vi "Update Data.vi"(0 "data in":T2, 1 "block size (elements)":i32, 2 "(empty) elements remaining":u32, 3 "command":refnum<notifier>, 4 "writing?":bool, 5 "error in (no error)":errorcluster, 8 "pending blocks in host buffer":i32) -> (14 "data out":T2, 15 "status":T1, 16 "preview size (elements)":i32, 17 "reopen file":bool, 18 "reopen total count (elements)":i64, 19 "error out":errorcluster)   [LabVIEW 2021, in "Disk Streaming.lvclass"]
doc: "Updates the disk streaming data with the transfer of a block, processes commands and prepares the status information.\n\nInputs:\n\n<B>data in</B>: Disk streaming data input.\n\n<B>block size (elements)</B>: The number of elements transferred in the block.\n\n<B>(empty) elements remaining</B>: When streaming from device to disk, set this input to the number of additional elements remaining in the host DMA buffer that are available for reading. When streaming from disk to device, set this input to the number of additional empty elements remaining in the host DMA buffer that are available for writing. This input is used only in the calculation of the Host DMA buffer utilization status.\n\n<B>command</B>: Reference to a notifier containing the last command.\n\n<B>writing?</B>: Set this input to true when streaming from device to disk, set this input to false when streaming from disk to device.\n\n<B>pending blocks in host buffer</B>: The number of the last blocks (including the current block transferring the <B>block size</B> elements) whose size is to be added to the Host DMA buffer utilization status. This input is used only in the calculation of the Host DMA buffer utilization status.\n\nOutputs:\n\n<B>data out</B>: Disk streaming data output.\n\n<B>status</B>: The disk streaming status. The status is not complete, this VI does not set the following elements in the status cluster: <B>Disk pending async operations</B> and <B>preview data</B>.\n\n<B>preview size (elements)</B>: The number of elements to use from the last block as the preview data.\n\n<B>reopen file</B>: A true on this output signals that the file should be reopened before reading the next block from it.\n\n<B>reopen total count (elements)</B>: The total number of elements to read from the file on a reopen to complete the streaming operation or until the next reopening of the file."
uses:
  Disk Streaming.lvclass
  Command.ctl
  Data.ctl
  Public/IO mode.ctl
  Status.ctl
  <vilib>/Utility/error.llb/Error Cluster From Error Code.vi
  <vilib>/ErrorRing/Error Ring.xnode
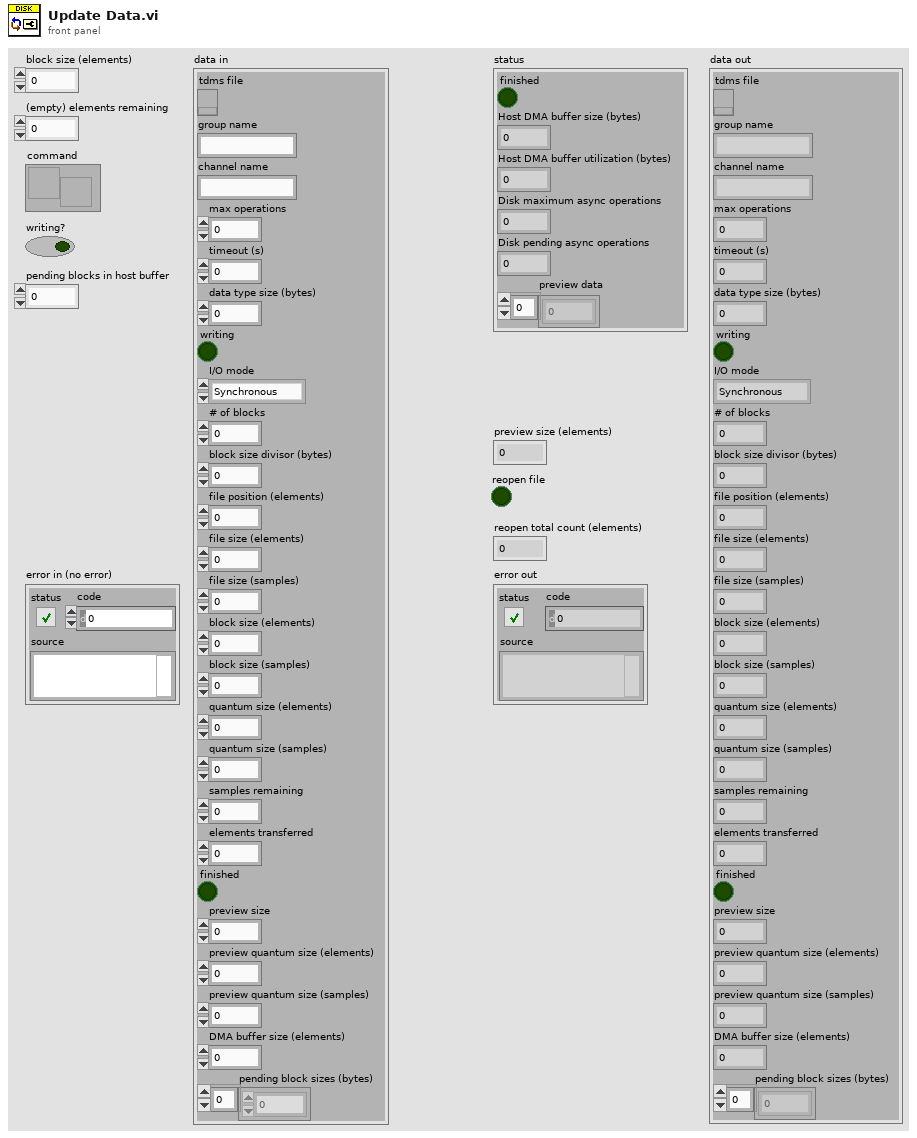
[diagram p1: front panel]
types:
  T1 = typedef "Disk Streaming.lvclass/Status.ctl" = cluster{"finished":bool, "Host DMA buffer size (bytes)":u64, "Host DMA buffer utilization (bytes)":u64, "Disk maximum async operations":u32, "Disk pending async operations":u32, "preview data":i16[]}
  T2 = typedef "Disk Streaming.lvclass/Data.ctl" = cluster{"tdms file":refnum<k34>, "group name":string, "channel name":string, "max operations":u32, "timeout (s)":dbl, "data type size (bytes)":u64, "writing":bool, "I/O mode":T3, "# of blocks":u32, "block size divisor (bytes)":u32, "file position (elements)":u64, "file size (elements)":i64, "file size (samples)":i64, "block size (elements)":u64, "block size (samples)":u64, "quantum size (elements)":u64, "quantum size (samples)":u64, "samples remaining":i64, "elements transferred":u64, "finished":bool, "preview size":i32, "preview quantum size (elements)":u64, "preview quantum size (samples)":u64, "DMA buffer size (elements)":u32, "pending block sizes (bytes)":u64[]}
  T3 = typedef "Disk Streaming.lvclass/IO mode.ctl" = enum16{"Synchronous", "Asynchronous", "Data Reference"}
  T4 = typedef "Disk Streaming.lvclass/Command.ctl" = cluster{"preview size":i32}
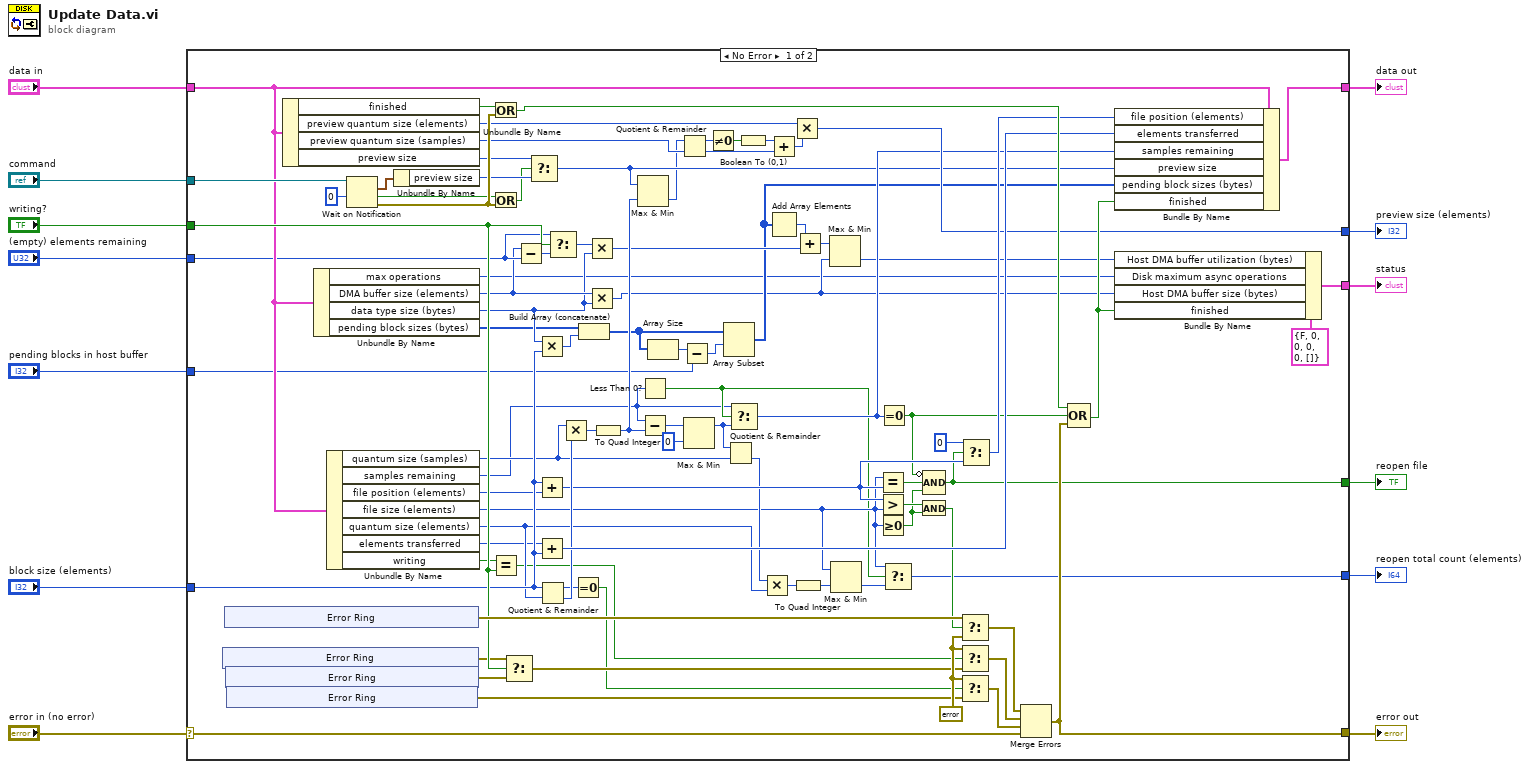
[diagram p0: block diagram]
diagram:
  n1 = case shown="No Error" "error in (no error)" {
    selector: "error in (no error)" -> [w78 w123]
    tunnel: "(empty) elements remaining" -> [w60 _]
    tunnel: "command" -> [w86 _]
    tunnel: [w83 w124] -> w11
    tunnel: "data in" -> [w61 w124]
    tunnel: [w89 w123] -> w8
    tunnel: "block size (elements)" -> [w44 _]
    tunnel: [w77 _] -> w6
    tunnel: "writing?" -> [w93 _]
    tunnel: [w63 _] -> w4
    tunnel: [w50 _] -> w3
    tunnel: "pending blocks in host buffer" -> [w41 _]
    tunnel: [w23 _] -> w1
    frame No Error {
      w101 = errorcluster {"status"=FALSE, "code"=0, "source"=""} ("t")
      n2 = xnode "Error Ring"() -> ("error out"=w88:errorcluster)
      n3 = xnode "Error Ring"() -> ("error out"=w100:errorcluster)
      n4 = xnode "Error Ring"() -> ("error out"=w87:errorcluster)
      n5 = xnode "Error Ring"() -> ("error out"=w99:errorcluster)
      n6 = Unbundle By Name(w61) -> ("finished"=w74:bool, "preview quantum size (elements)"=w51:u64, "preview quantum size (samples)"=w52:u64, "preview size"=w73:i32)
      n7 = Unbundle By Name(w61) -> ("max operations"=w14:u32, "DMA buffer size (elements)"=w58:u32, "data type size (bytes)"=w45:u64, "pending block sizes (bytes)"=w38:u64[])
      n8 = Unbundle By Name(w61) -> ("quantum size (samples)"=w31:u64, "samples remaining"=w18:i64, "file position (elements)"=w21:u64, "file size (elements)"=w25:i64, "quantum size (elements)"=w29:u64, "elements transferred"=w19:u64, "writing"=w20:bool)
      n9 = Wait on Notification(notifier=w86, timeout in ms (-1)=0) -> (notification=w84:T4, timed out?=w48:bool, error out=w95:errorcluster)  [unwired: 2 in, 1 out]
      n10 = Unbundle By Name(w84) -> ("preview size"=w72:i32)
      n11 = Or(x=w74, y=w95) -> (x .or. y?=w97:bool)
      n12 = Or(x=w48, y=w95) -> (x .or. y?=w47:bool)
      n13 = Equal?(x=w20, y=w93) -> (x = y?=w22:bool)
      n14 = Select(t=w88, s=w93, f=w87) -> (s? t:f=w98:errorcluster)
      n15 = Subtract(x=w58, y=w60) -> (x-y=w62:u32)
      n16 = Select(t=w73, s=w47, f=w72) -> (s? t:f=w16:i32)
      n17 = Multiply(x=w45, y=w44) -> (x*y=w43:u64)
      n18 = Add(x=w44, y=w21) -> (x+y=w68:u64)
      n19 = Add(x=w19, y=w44) -> (x+y=w94:u64)
      n20 = Quotient & Remainder(x=w44, y=w29) -> (x-y*floor(x/y)=w65:u64, floor(x/y)=w82:u64)
      n21 = Select(t=w60, s=w93, f=w62) -> (s? t:f=w59:u32)
      n22 = Multiply(x=w31, y=w82) -> (x*y=w17:u64)
      n23 = Equal To 0?(x=w65) -> (x = 0?=w91:bool)
      n24 = Build Array (concatenate)(w38, w43) -> (w39:u64[])
      n25 = Multiply(x=w59, y=w45) -> (x*y=w49:u64)
      n26 = Multiply(x=w58, y=w45) -> (x*y=w33:u64)
      n27 = To Quad Integer(1:w17) -> (0:w102:i64)
      n28 = Max & Min(x=w16, y=w102) -> (min(x,y)=w15:i64)  [unwired: 1 out]
      n29 = Less Than 0?(x=w18) -> (x < 0?=w24:bool)
      n30 = Subtract(x=w18, y=w102) -> (x-y=w81:i64)
      n31 = Array Size(array=w39) -> (size(s)=w42:i32)
      n32 = Quotient & Remainder(x=w15, y=w52) -> (x-y*floor(x/y)=w53:u64, floor(x/y)=w56:u64)
      n33 = Subtract(x=w42, y=w41) -> (x-y=w40:i32)
      n34 = Max & Min(x=w81, y=i64 0) -> (max(x,y)=w32:i64)  [unwired: 1 out]
      n35 = Not Equal To 0?(x=w53) -> (x != 0?=w54:bool)
      n36 = Array Subset(array=w39, index=w40) -> (w37:u64[])  [unwired: 1 in]
      n37 = Quotient & Remainder(x=w32, y=w31) -> (floor(x/y)=w30:u64)  [unwired: 1 out]
      n38 = Select(t=w18, s=w24, f=w32) -> (s? t:f=w46:i64)
      n39 = Boolean To (0,1)(Boolean=w54) -> (0, 1=w55:i16)
      n40 = Multiply(x=w30, y=w29) -> (x*y=w28:u64)
      n41 = Add(x=w55, y=w56) -> (x+y=w57:u64)
      n42 = Add Array Elements(numeric array=w37) -> (sum=w36:u64)
      n43 = Multiply(x=w51, y=w57) -> (x*y=w50:u64)
      n44 = To Quad Integer(1:w28) -> (0:w27:i64)
      n45 = Add(x=w36, y=w49) -> (x+y=w34:u64)
      n46 = Max & Min(x=w34, y=w33) -> (min(x,y)=w35:u64)  [unwired: 1 out]
      n47 = Max & Min(x=w25, y=w27) -> (min(x,y)=w26:i64)  [unwired: 1 out]
      n48 = Equal?(x=w25, y=w68) -> (x = y?=w71:bool)
      n49 = Greater?(x=w68, y=w25) -> (0:w70:bool)
      n50 = Greater Or Equal To 0?(x=w25) -> (x >= 0?=w69:bool)
      n51 = Equal To 0?(x=w46) -> (x = 0?=w64:bool)
      n52 = Select(t=w25, s=w24, f=w26) -> (s? t:f=w23:i64)
      n53 = And(x=w70, y=w69) -> (x .and. y?=w90:bool)
      n54 = Compound Arithmetic op=AND(invert w64, w71, w69) -> (w63:bool)
      n55 = Select(t=w100, s=w90, f=w101) -> (s? t:f=w66:errorcluster)
      n56 = Select(t=w101, s=w22, f=w98) -> (s? t:f=w76:errorcluster)
      n57 = Select(t=w101, s=w91, f=w99) -> (s? t:f=w75:errorcluster)
      n58 = Select(t=u64 0, s=w63, f=w68) -> (s? t:f=w92:u64)
      n59 = Merge Errors(w66, w76, w75, w78) -> (w89:errorcluster)
      n60 = Compound Arithmetic op=OR(w97, w64, w89) -> (w96:bool)
      n61 = Bundle By Name(cluster=w61, "file position (elements)"=w92, "elements transferred"=w94, "samples remaining"=w46, "preview size"=w16, "pending block sizes (bytes)"=w37, "finished"=w96) -> (w83:T2)
      n62 = Bundle By Name(cluster=T1 {"finished"=FALSE, "Host DMA buffer size (bytes)"=0, "Host DMA buffer utilization (bytes)"=0, "Disk maximum async operations"=0, "Disk pending async operations"=0, "preview data"=[]} ("Disk Streaming Descriptor Status"), "Host DMA buffer utilization (bytes)"=w35, "Disk maximum async operations"=w14, "Host DMA buffer size (bytes)"=w33, "finished"=w96) -> (w77:T1)
    }
    frame Error {
    }
  }
  "error out" <- w8
  "data out" <- w11
  "status" <- w6
  "reopen file" <- w4
  "preview size (elements)" <- w3
  "reopen total count (elements)" <- w1
